vi "Active Plugins.vi"(8 "error in (no error)":errorcluster, 11 "Framework in":refnum<class "Framework.lvclass">) -> (0 "error out":errorcluster, 3 "Framework out":refnum<class "Framework.lvclass">)   [LabVIEW 2021, in "DSF Core.lvlib" / "Framework.lvclass"]
uses:
  Framework.lvclass
  Framework.lvclass/Framework.ctl
  Plugin/Plugin.lvclass/Plugin.ctl
  Timing/Timing.lvclass/Timing.ctl
  Transfer Group/Transfer Group.lvclass/Transfer Group.ctl
  Timing/Is Active Cycle.vi
  Plugin/Iteration.vi
  Timing/Get Decimation.vi
  Timing/Get Offset.vi
  Plugin/Get Timing.vi
  Timing/Get Iteration.vi
  Plugin/Plugin.lvclass
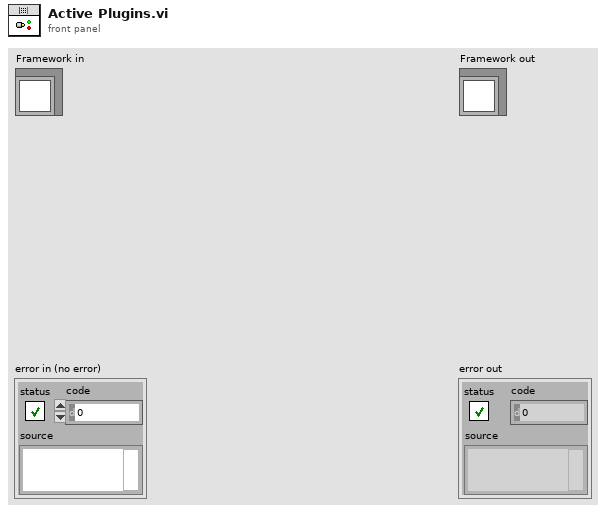
[diagram p1: front panel]
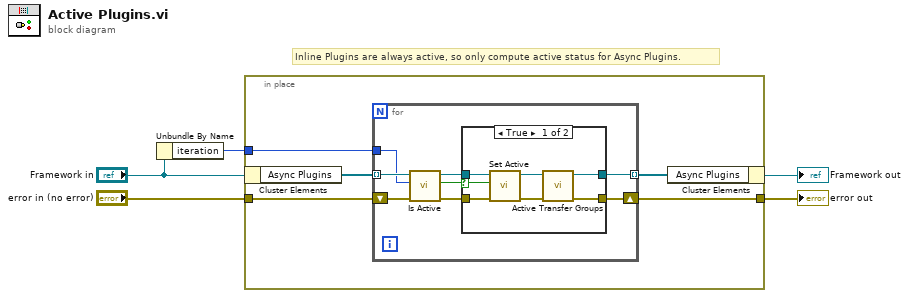
[diagram p0: block diagram]
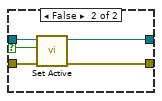
[diagram p2: hidden frame]
diagram:
  # "Inline Plugins are always active, so only compute active status for Async Plugins."
  n1 = Unbundle By Name("Framework in") -> ("iteration"=w3:u64)
  n2 = in-place {
    in-place-border: w3 -> [w8]
    in-place-border: [w7] -> w1
    in-place-border: "error in (no error)" -> [w6]
    n3 = in-place-cluster #1("Framework in") -> ("Async Plugins"=w10:refnum<class "Plugin.lvclass">[])
    n4 = for {
      tunnel: w10 -> [w17] mode=indexing
      tunnel: [w15] -> w9 mode=indexing
      tunnel: w8 -> [w14]
      shift-right: [w13] -> w7
      shift-left: w6 -> [w11]
      n5 = call "Is Active.vi"("cycle count"=w14, "Plugin in"=w17) -> ("active this cycle?"=w12:bool, "Plugin out"=w16:refnum<class "Plugin.lvclass">)  [unwired: 8 in]
      n6 = case shown="True" w12 {
        selector: w12 -> [w19 w25]
        tunnel: w16 -> [w23 w27]
        tunnel: [w21 w26] -> w15
        tunnel: [w20 w24] -> w13
        tunnel: w11 -> [w18 w24]
        frame True {
          n7 = call "Set Active.vi"("active"=w19, "Plugin in"=w23) -> ("Plugin out"=w22:refnum<class "Plugin.lvclass">)  [unwired: 9 in]
          n8 = call "Active Transfer Groups.vi"("error in (no error)"=w18, "Plugin in"=w22) -> ("error out"=w20:errorcluster, "Plugin out"=w21:refnum<class "Plugin.lvclass">)  [unwired: 8 in]
        }
        frame False {
          n9 = call "Set Active.vi"("active"=w25, "Plugin in"=w27) -> ("Plugin out"=w26:refnum<class "Plugin.lvclass">)  [unwired: 9 in]
        }
      }
    }
    n10 = in-place-cluster #1("Async Plugins"=w9) -> (→"Framework out":refnum<class "Framework.lvclass">)
  }
  "error out" <- w1
